vi "Active collect.vi"(11 "MechanismMetrics in":T1) -> ()   [LabVIEW 2014]
uses:
  MechanismMetrics.ctl
  Lifter States.ctl
  Auto Lifter States.ctl
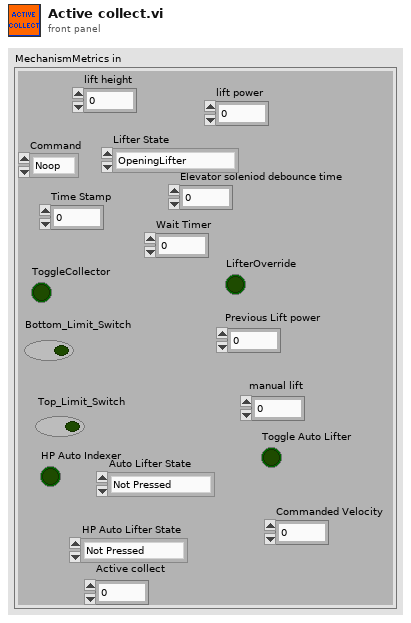
[diagram p1: front panel]
types:
  T1 = typedef "MechanismMetrics.ctl" = cluster{"lift height":dbl, "Command":enum16{"Noop", "Flagged"}, "Time Stamp":u32, "ToggleCollector":bool, "Bottom_Limit_Switch ":bool, "Top_Limit_Switch":bool, "lift power":dbl, "Elevator soleniod debounce time   ":dbl, "LifterOverride":bool, "Previous Lift power":dbl, "manual lift":dbl, "Lifter State":T2, "Auto Lifter State":T3, "Toggle Auto Lifter":bool, "Wait Timer":dbl, "HP Auto Indexer":bool, "HP Auto Lifter State":T3, "Commanded Velocity":dbl, "\nActive collect":dbl}
  T2 = typedef "Lifter States.ctl" = enum16{"OpeningLifter", "LifterOpen", "ClosingLifter", "LifterClosed"}
  T3 = typedef "Auto Lifter States.ctl" = enum16{"Not Pressed", "THE_END", "WAIT_FOR_RELEASE", "Press Detected", "To Release Stacked1", "To Collect", "Open Lifter", "WAIT", "Close", "To Stack1"}
  T4 = typedef "WPI_MotorControlDeviceRef.ctl" = cluster{"DeviceStatus":errorcluster, "Type":T5, "PWM":cluster{"Controller":T6, "PWM Channel":T7, "DeadBand":T8}, "CAN":cluster{"Device Number":u8, "Control Mode":T9, "Semaphore":T10, "Max Vout":dbl, "TalonSRX Control Mode":T11}, "Invert":bool, "TransformRef":T12, "InvTransformRef":T12}
  T5 = typedef "WPI_MotorControlType.ctl" = enum16{"PWM", "CAN", "CANTalonSRX"}
  T6 = typedef "FPGA_TypedefDigitalModule.ctl" = enum16{"Controller 1"}
  T7 = typedef "FPGA_DIOPWMChannel.ctl" = enum8{"PWM 0", "PWM 1", "PWM 2", "PWM 3", "PWM 4", "PWM 5", "PWM 6", "PWM 7", "PWM 8", "PWM 9", "PWM MXP 0", "PWM MXP 1", "PWM MXP 2", "PWM MXP 3", "PWM MXP 4", "PWM MXP 5", "PWM MXP 6", "PWM MXP 7", "PWM MXP 8", "PWM MXP 9", "Invalid"}
  T8 = typedef "WPI_PWMDeadband.ctl" = cluster{"Name":string, "maxPositivePwm":i32, "minPositivePwm":i32, "centerPwm":i32, "maxNegativePwm":i32, "minNegativePwm":i32, "angularRange":u16}
  T9 = typedef "WPI_CANJaguar_ControlMode.ctl" = enum8{"Percent VBus", "Current", "Speed", "Position", "Voltage"}
  T10 = typedef "Semaphore RefNum" = refnum<k1>
  T11 = typedef "WPI_CANTalonSRX_APIControlMode.ctl" = enum8{"Percent VBus", "Speed", "Position", "Slave", "Unchanged / Invalid"}
  T12 = typedef "WPI_PWMTransform_ConPane.ctl" = refnum<vi>
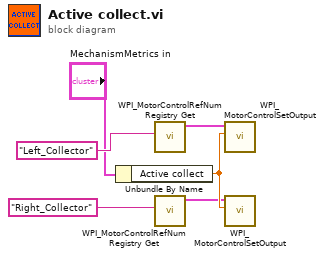
[diagram p0: block diagram]
diagram:
  n1 = Unbundle By Name("MechanismMetrics in") -> ("Active collect"=w6:dbl)
  n2 = call <vilib>:"WPI_MotorControlRefNum Registry Get.vi"("refnum name"="Left_Collector") -> ("MotorControlDevRef"=w5:T4)  [unwired: 9 in, 1 out]
  n3 = call <vilib>:"WPI_MotorControlRefNum Registry Get.vi"("refnum name"="Right_Collector") -> ("MotorControlDevRef"=w4:T4)  [unwired: 9 in, 1 out]
  n4 = call <vilib>:"WPI_MotorControlSetOutput.vi"("Output"=w6, "MotorControlDevRef"=w5) -> ()  [unwired: 7 in, 3 out]
  n5 = call <vilib>:"WPI_MotorControlSetOutput.vi"("Output"=w6, "MotorControlDevRef"=w4) -> ()  [unwired: 7 in, 3 out]
